vi "Open Reference.vi"(8 "error in (no error)":errorcluster, 11 "Item in":refnum<class "Item.lvclass">) -> (0 "error out":errorcluster, 3 "Item out":refnum<class "Item.lvclass">)   [LabVIEW 2020, in "Code Cleanup.lvlib" / "Item.lvclass"]
uses:
  Item.lvclass
  Item.lvclass/Item.ctl
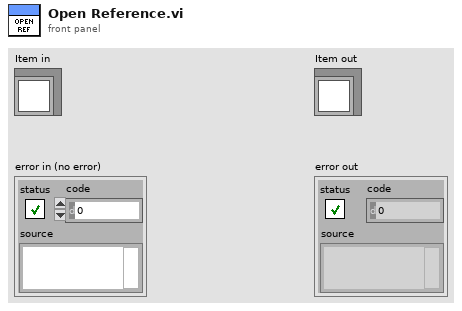
[diagram p1: front panel]
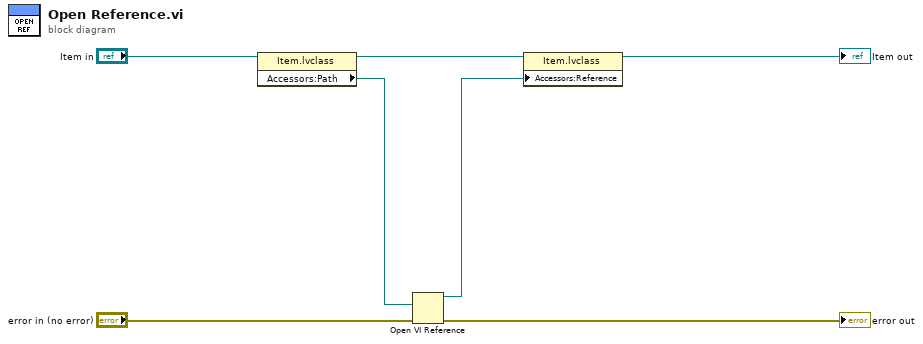
[diagram p0: block diagram]
diagram:
  n1 = property class="Item.lvclass"(reference="Item in") -> (reference out=w5:refnum<class "Item.lvclass">, "Accessors:Path"=w3:path)  [unwired: 1 in, 1 out]
  n2 = Open VI Reference(vi path=w3, error in (no error)="error in (no error)") -> (vi reference=w2:refnum<vi>, error out=→"error out":errorcluster)  [unwired: 4 in]
  n3 = property class="Item.lvclass"(reference=w5, "Accessors:Reference"=w2) -> (reference out=→"Item out":refnum<class "Item.lvclass">)  [unwired: 1 in, 1 out]
